vi "check_finalMovimiento.vi"(8 "error in (no error)":errorcluster, 9 "Cluster_Tracking in":T2, 10 "Enum in":T1, 11 "VISA Refnum in":refnum<visa-resource-name>) -> (0 "error out":errorcluster, 1 "Cluster_Tracking out":T2, 2 "Enum out":T1, 3 "VISA Refnum out":refnum<visa-resource-name>, 4 "Movimiento realizado?":bool)   [LabVIEW 2019]
uses:
  Typedefs/Cluster_tracking.ctl
  Typedefs/Tipo_movimiento.ctl
  Typedefs/Comandos.ctl
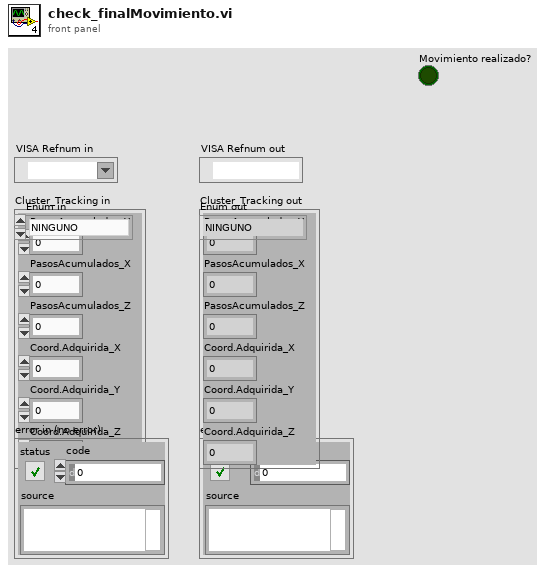
[diagram p1: front panel]
types:
  T1 = typedef "Tipo_movimiento.ctl" = enum16{"NINGUNO", "AVANZAR", "RETROCEDER", "DERECHA", "IZQUIERDA", "SUBIRZ", "BAJARZ", "HOME", "HOME_Z"}
  T2 = typedef "Cluster_tracking.ctl" = cluster{"PasosAcumulados_Y":i32, "PasosAcumulados_X":i32, "PasosAcumulados_Z":i32, "Coord.Adquirida_X":i32, "Coord.Adquirida_Y":i32, "Coord.Adquirida_Z":i32}
  T3 = typedef "Comandos.ctl" = enum16{"H", "FH", "FM", "FI", "FX", "FY", "FZ", "I", "OK"}
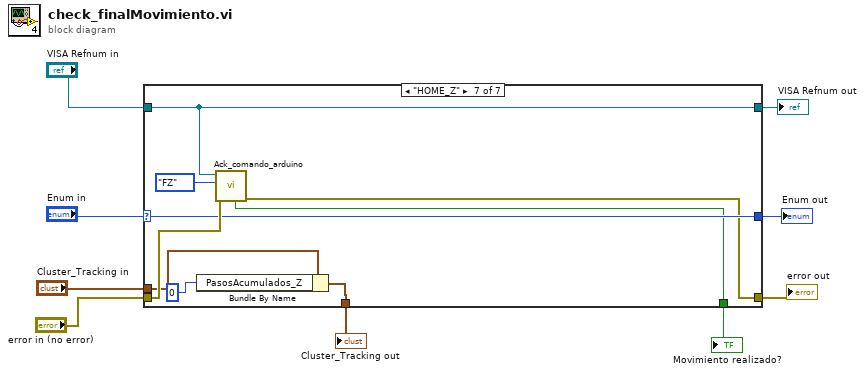
[diagram p0: block diagram]
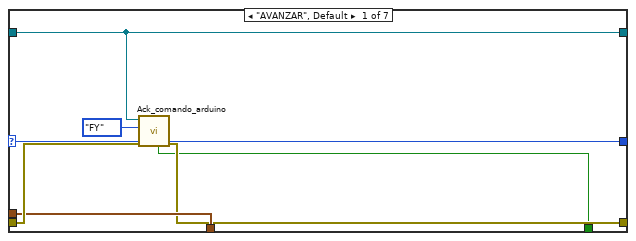
[diagram p2: hidden frame]
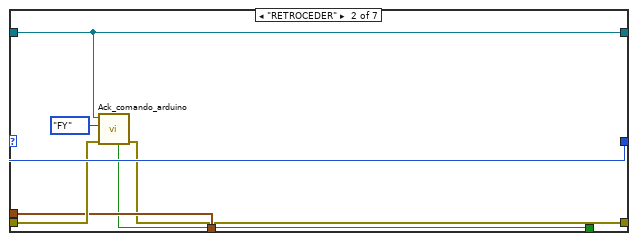
[diagram p3: hidden frame]
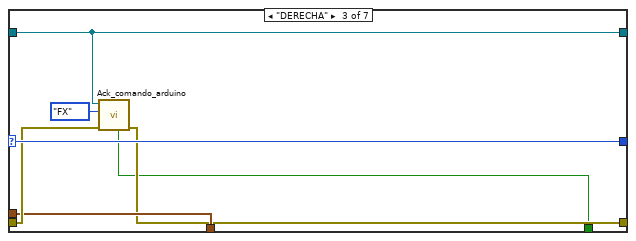
[diagram p4: hidden frame]
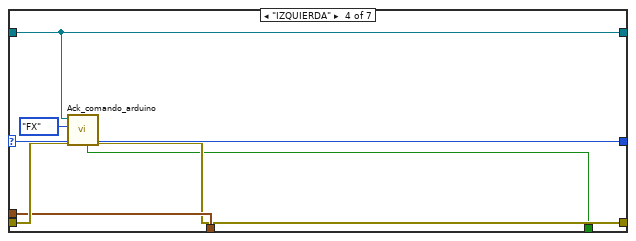
[diagram p5: hidden frame]
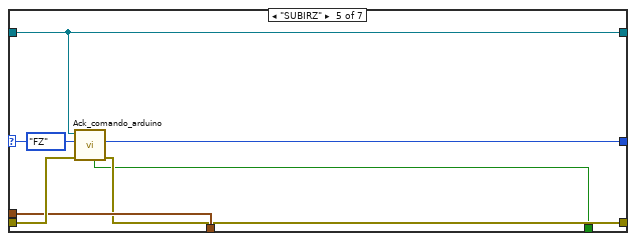
[diagram p6: hidden frame]
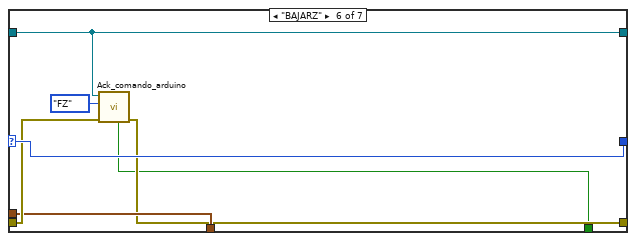
[diagram p7: hidden frame]
diagram:
  n1 = case shown="\"HOME_Z\"" "Enum in" {
    selector: "Enum in" -> [w13 w22 w29 w36 w43 w50 w57]
    tunnel: [w15 w20 w27 w34 w41 w48 w58] -> w3
    tunnel: "VISA Refnum in" -> [w15 w20 w27 w34 w41 w48 w58]
    tunnel: "error in (no error)" -> [w14 w21 w28 w35 w42 w49 w59]
    tunnel: [w11 w18 w25 w32 w39 w46 w53] -> w9
    tunnel: [w13 w22 w29 w36 w43 w50 w57] -> w6
    tunnel: "Cluster_Tracking in" -> [w12 w19 w26 w33 w40 w47 w56]
    tunnel: [w12 w19 w26 w33 w40 w47 w54] -> w8
    tunnel: [w10 w17 w24 w31 w38 w45 w52] -> w1
    frame "AVANZAR", Default {
      n2 = call "Ack_comando_arduino.vi"("error in (no error)"=w14, 10:Comandos."FY", "VISA resource name"=w15) -> ("error IO"=w11:errorcluster, "Movimiento realizado?"=w10:bool)  [unwired: 6 in, 1 out]
    }
    frame "RETROCEDER" {
      n3 = call "Ack_comando_arduino.vi"("error in (no error)"=w21, 10:Comandos."FY", "VISA resource name"=w20) -> ("error IO"=w18:errorcluster, "Movimiento realizado?"=w17:bool)  [unwired: 6 in, 1 out]
    }
    frame "DERECHA" {
      n4 = call "Ack_comando_arduino.vi"("error in (no error)"=w28, 10:Comandos."FX", "VISA resource name"=w27) -> ("error IO"=w25:errorcluster, "Movimiento realizado?"=w24:bool)  [unwired: 6 in, 1 out]
    }
    frame "IZQUIERDA" {
      n5 = call "Ack_comando_arduino.vi"("error in (no error)"=w35, 10:Comandos."FX", "VISA resource name"=w34) -> ("error IO"=w32:errorcluster, "Movimiento realizado?"=w31:bool)  [unwired: 6 in, 1 out]
    }
    frame "SUBIRZ" {
      n6 = call "Ack_comando_arduino.vi"("error in (no error)"=w42, 10:Comandos."FZ", "VISA resource name"=w41) -> ("error IO"=w39:errorcluster, "Movimiento realizado?"=w38:bool)  [unwired: 6 in, 1 out]
    }
    frame "BAJARZ" {
      n7 = call "Ack_comando_arduino.vi"("error in (no error)"=w49, 10:Comandos."FZ", "VISA resource name"=w48) -> ("error IO"=w46:errorcluster, "Movimiento realizado?"=w45:bool)  [unwired: 6 in, 1 out]
    }
    frame "HOME_Z" {
      n8 = Bundle By Name(cluster=w56, "PasosAcumulados_Z"=0) -> (w54:T2)
      n9 = call "Ack_comando_arduino.vi"("error in (no error)"=w59, 10:Comandos."FZ", "VISA resource name"=w58) -> ("error IO"=w53:errorcluster, "Movimiento realizado?"=w52:bool)  [unwired: 6 in, 1 out]
    }
  }
  "error out" <- w9
  "Cluster_Tracking out" <- w8
  "Enum out" <- w6
  "VISA Refnum out" <- w3
  "Movimiento realizado?" <- w1
